vi "getApi.vi"(8 "error in (no error)":errorcluster, 11 "YoutuberDownloader in":refnum<class "YoutuberDownloader.lvclass">) -> (0 "error out":errorcluster, 2 "ThirdPartyYoutubeLib.lvclass":refnum<class "ThirdPartyYoutubeLib.lvclass">, 3 "YoutuberDownloader out":refnum<class "YoutuberDownloader.lvclass">)   [LabVIEW 2017, in "YoutuberDownloader.lvclass"]
uses:
  YoutuberDownloader.lvclass
  ThirdPartyYoutubeLib Class/ThirdPartyYoutubeLib.lvclass
  YoutuberDownloader.lvclass/YoutuberDownloader.ctl
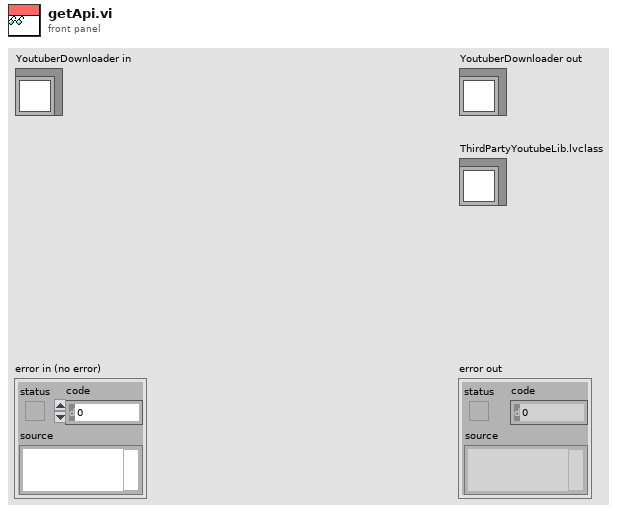
[diagram p1: front panel]
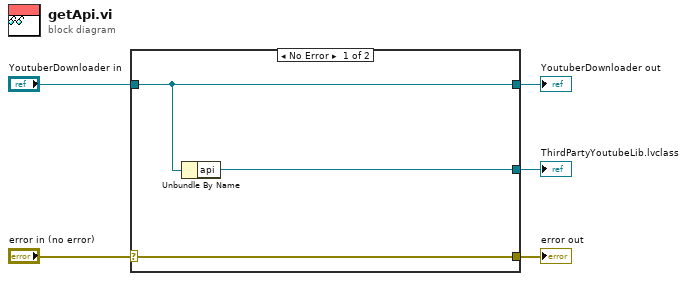
[diagram p0: block diagram]
diagram:
  n1 = case shown="No Error" "error in (no error)" {
    selector: "error in (no error)" -> [w8 w9]
    tunnel: [w8 w9] -> w4
    tunnel: [w7 w10] -> w2
    tunnel: "YoutuberDownloader in" -> [w7 w10]
    tunnel: [w6 _] -> w1
    frame No Error {
      n2 = Unbundle By Name(w7) -> ("api"=w6:refnum<class "ThirdPartyYoutubeLib.lvclass">)
    }
    frame Error {
    }
  }
  "error out" <- w4
  "YoutuberDownloader out" <- w2
  "ThirdPartyYoutubeLib.lvclass" <- w1
